vi "dataProcess_coherenceLength.vi"(0 "reference":refnum<class "OSA.lvclass">, 1 "samplesPerRefPeriod":i32, 2 "interferogram":sgl[](array[numeric]), 3 "X min interferogram (cm)":sgl, 4 "X max interferogram (cm)":sgl, 5 "error in (no error)":errorcluster, 6 "X range":T1(ring), 8 "X min (cm)":sgl format="%.2f", 10 "X max (cm)":sgl format="%.2f") -> (14 "duplicate reference":refnum<class "OSA.lvclass">, 15 "coherence length error(cm)":dbl, 16 "coherence length (cm)":dbl, 19 "error out":errorcluster)   [LabVIEW 2010, in "OSA.lvclass"]
doc: "Estimates the coherence length of the input light source by analyzing the interferogram.\n\nThis vi calls FTS_CoherenceLength_Array, (FTSLib.dll), with the interferogram input parameter pointing to the interferogram control data of this vi or, if empty, to the labview interferogram buffer. \n\nSee buffer_get.vi or trace_toLVBuffer.vi for OSA200 labview buffer handling."
uses:
  OSA.lvclass
  FTSLib.dll
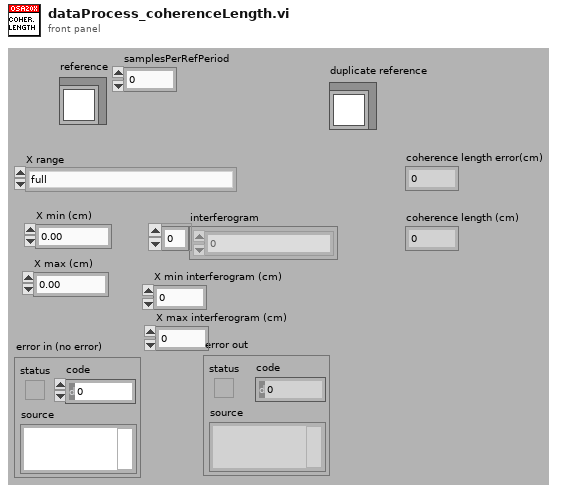
[diagram p1: front panel]
types:
  T1 = enum16{"full", "zero symmetric (-X min .... +X min)", "zero asymmetric (X min .... X max)"}
  T2 = cluster{"length":u32, "X min (cm)":sgl, "X max (cm)":sgl, "saturated":bool, "broadband":bool, "isMonoChromatic":bool, "peakToPeak, (counts)":dbl, "peakToPeak position (cm)":dbl, "samplesPerRefPeriod":i32}
  T3 = enum16{"get", "init", "set interferogram", "set spectrum", "cleanUp"}
  T4 = typedef "OSA.lvclass/ObjectAttributes.ctl" = cluster{"Stop":bool, "dataType":T5, "spectrometerIdx":u16, "buffer size interferogram":i32, "interferogram":cluster{"new":bool, "plot_x_ min":sgl, "plot_x_max":sgl, "plot_y_min":sgl, "plot_y_max":sgl, "Graph Intrfrgrm":T6, "timeStamp":u32, "signal (%)":dbl, "traces":cluster{"idx":u32, "broadBand":bool, "monoChromatic":bool, "peakToPeakSignal":dbl, "peakToPeakPos":dbl}[], "traces idx last":i32}, "spectrum":cluster{"new":bool, "plot_x_min":sgl, "plot_x_max":sgl, "plot_unit_x":T7, "plot_unit_y":T8, "plot_y_min":sgl, "plot_y_max":sgl, "Graph Spectrum":T6, "timeStamp":u32, "X_VAL_OPTIONS":enum16{"MIN_MAX", "ARRAY"}, "traces":cluster{"idx":u32}[], "traces idx last":i32}, "Thorlabs_OSA_64.lvclass:queue_action.ctlqueue ref":refnum<queue>, "action":T9, "plot zoom step":dbl, "buffer semaphore":T10, "acq stopped":bool, "dataType active":T5, "temperature (degr C)":sgl, "pressure (hPa)":sgl, "rel humidity (%)":sgl, "settings":cluster{"resolution":T11, "sensitivity":T12, "Average":bool, "average nr":u32, "apodisation":T13, "acq delay (ms)":u32, "airMesure":T14, "wmtr on":bool, "intfgrm_smooth_width":u16, "intfgrm_smooth_nrOfPasses":u16, "intfgrm_smooth":T15, "phaseCorrection":T16, "zeroFill":u8, "spectr_smooth":T15, "spectr_smooth_width":u16, "spectr_smooth_nrOfPasses":u16, "resolution (/cm)":sgl, "REF wavelength, (nm)":dbl, "gain_idx":u16, "gainAuto":bool, "gain_relative":dbl, "PD sensitivity mode":T17, "PD senseMode implemented":bool, "SensorTemperature implemented":bool, "SensorPressure implemented":bool, "SensorHumidity implemented":bool}, "peaks position":sgl[], "peaks width":sgl[], "peaks height":sgl[], "peaks max nr":u32, "peaks latest nr":i32, "peaks new":bool, "power":dbl, "power new":bool, "path":string, "wavelength (WNr)":dbl, "wavelength new":bool, "buffer size spectrum":i32, "status":string, "VI reference":refnum<vi>, "funcPointer":u64, "libraryPointer":u64, "singleAcquisition":bool, "coherenceLength (cm)":dbl, "coherenceLength new":bool, "spectrometer model":string, "spectrometer serial nr":string, "peaks thld left":sgl[], "peaks thld right":sgl[], "coherenceLength error (cm)":dbl, "ADC bits":u16, "peaks position centroid":sgl[], "peaks height centroid":sgl[], "OSA series":T18, "channel index (all)":u16}
  T5 = typedef "OSA.lvclass/acq_dataType.ctl" = enum16{"none", "interferogram", "spectrum"}
  T6 = typedef "OSA.lvclass/graph_intensity.ctl" = refnum<vi>
  T7 = typedef "OSA.lvclass/spectrum_x_unit.ctl" = enum16{"wavenr/cm", "THz", "eV", "nm_air", "nm_vac"}
  T8 = typedef "OSA.lvclass/y_unit.ctl" = enum16{"ADC counts", "dBm pwr absolute", "dBm pwr density", "mW pwr absolute", "mW pwr density"}
  T9 = typedef "OSA.lvclass/queue_action.ctl" = enum16{"none", "stop", "GUI_plotInterferogram", "GUI_plotSpectrum", "GUI_plotInterferogramRescale", "GUI_plotSpectrumRescale", "GUI_plotInterferogramReset", "GUI_plotSpectrumReset", "GUI_plotInterferogramAutoScaleY", "GUI_plotSpectrumAutoScaleY", "GUI_plotInterferogramZoomOut", "GUI_plotSpectrumZoomOut", "GUI_plotInterferogramPane", "GUI_plotSpectrumPane", "GUI_plotInterferogramZoomMouse", "GUI_plotSpectrumZoomMouse", "ENVIRONMENT temperature", "ENVIRONMENT pressure", "MODE_resolution set", "MODE_resolution get", "MODE_sensitivity set", "MODE_sensitivity get", "MODE_PDTemperature set", "MODE_PDTemperature get", "REBOOT/RESET firmware", "ACQASYNC_acquireSingleSpectrum", "ACQASYNC_continuous start", "ACQASYNC_continuous stop\n", "ACQASYNC_get last interferogram", "ACQASYNC_get last spectrum", "ACQASYNC_get last waveNr", "ACQOPT_interferogram smoothing set", "ACQOPT_interferogram smoothing get", "ACQOPT_spectrum smoothing set", "ACQOPT_spectrum smoothing get", "ACQOPT_apodisation type set", "ACQOPT_apodisation type get", "ACQOPT_phase correction type set", "ACQOPT_phase correction type get", "ACQOPT_acqIntervall_set", "ACQOPT_acqIntervall_get", "ACQOPT_average spectrum set", "ACQOPT_average spectrum get", "ACQOPT_rolling average set", "ACQOPT_rolling average get", "ACQOPT_zero fill factor set", "ACQOPT_zero fill factor get", "ACQOPT_cycle counting set", "ACQOPT_cycle counting get", "ACQOPT_air measure option set", "ACQOPT_air measure option get", "ACQOPT_gainLevel auto get", "ACQOPT_gainLevel auto set", "ACQOPT_gainLevel get", "ACQOPT_gainLevel set", "ACQOPT_getAll", "INSTRUMENT_PROPERTY_range_WaveNr_min", "INSTRUMENT_PROPERTY_range_WaveNr_max", "INSTRUMENT_PROPERTY_reference_wavelength_cm^-1", "INSTRUMENT_PROPERTY_samplesPerRefPeriod", "INSTRUMENT_PROPERTY_resolution_waveNrPercm", "INSTRUMENT_PROPERTY_availableGainLevels", "INSTRUMENT_PROPERTY_status", "CONVERT", "ANALYSE_POWER", "ANALYSE_PEAKS", "ANALYSE_WAVELENGTH", "ANALYSE_SPECTRUM", "ANALYSE_INTERFEROGRAM", "ANALYSE_COHERENCE_LENGTH", "MATH", "MATH_power", "MATH_peaks", "FILE", "miscellaneous"}
  T10 = typedef "Semaphore RefNum" = refnum<k1>
  T11 = typedef "OSA.lvclass/resolution.ctl" = enum16{"low", "high"}
  T12 = typedef "OSA.lvclass/sensitivityMode.ctl" = enum16{"low", "low medium", "high medium", "high"}
  T13 = typedef "OSA.lvclass/apodisation.ctl" = enum16{"NONE", "NORTON_BEER_WEAK", "NORTON_BEER_MEDIUM", "NORTON_BEER_STRONG", "TRIANGULAR", "COSINE", "HANN", "HAMMING", "BLACKMANHARRIS3", "BLACKMANHARRIS4", "GAUSSIAN"}
  T14 = typedef "OSA.lvclass/airMeasure.ctl" = enum16{"TEMPERATURE", "PRESSURE"}
  T15 = typedef "OSA.lvclass/smoothing.ctl" = enum16{"NONE", "BINOMIAL", "SAVITSKY_GOLAY", "FOURIER", "MOVING_AVERAGE", "GAUSSIAN"}
  T16 = typedef "OSA.lvclass/phaseCorrection.ctl" = enum16{"NONE", "MERTZ", "FORMAN", "MERTZ_FILE", "FORMAN_FILE", "FUTURE COMP."}
  T17 = typedef "OSA.lvclass/PDTemperatureMode.ctl" = enum16{"cool: better sensitivity/noise floor", "warm: extended wl range"}
  T18 = typedef "OSA_series.ctl" = enum16{"OSA200", "OSA300", "UNKNOWN"}
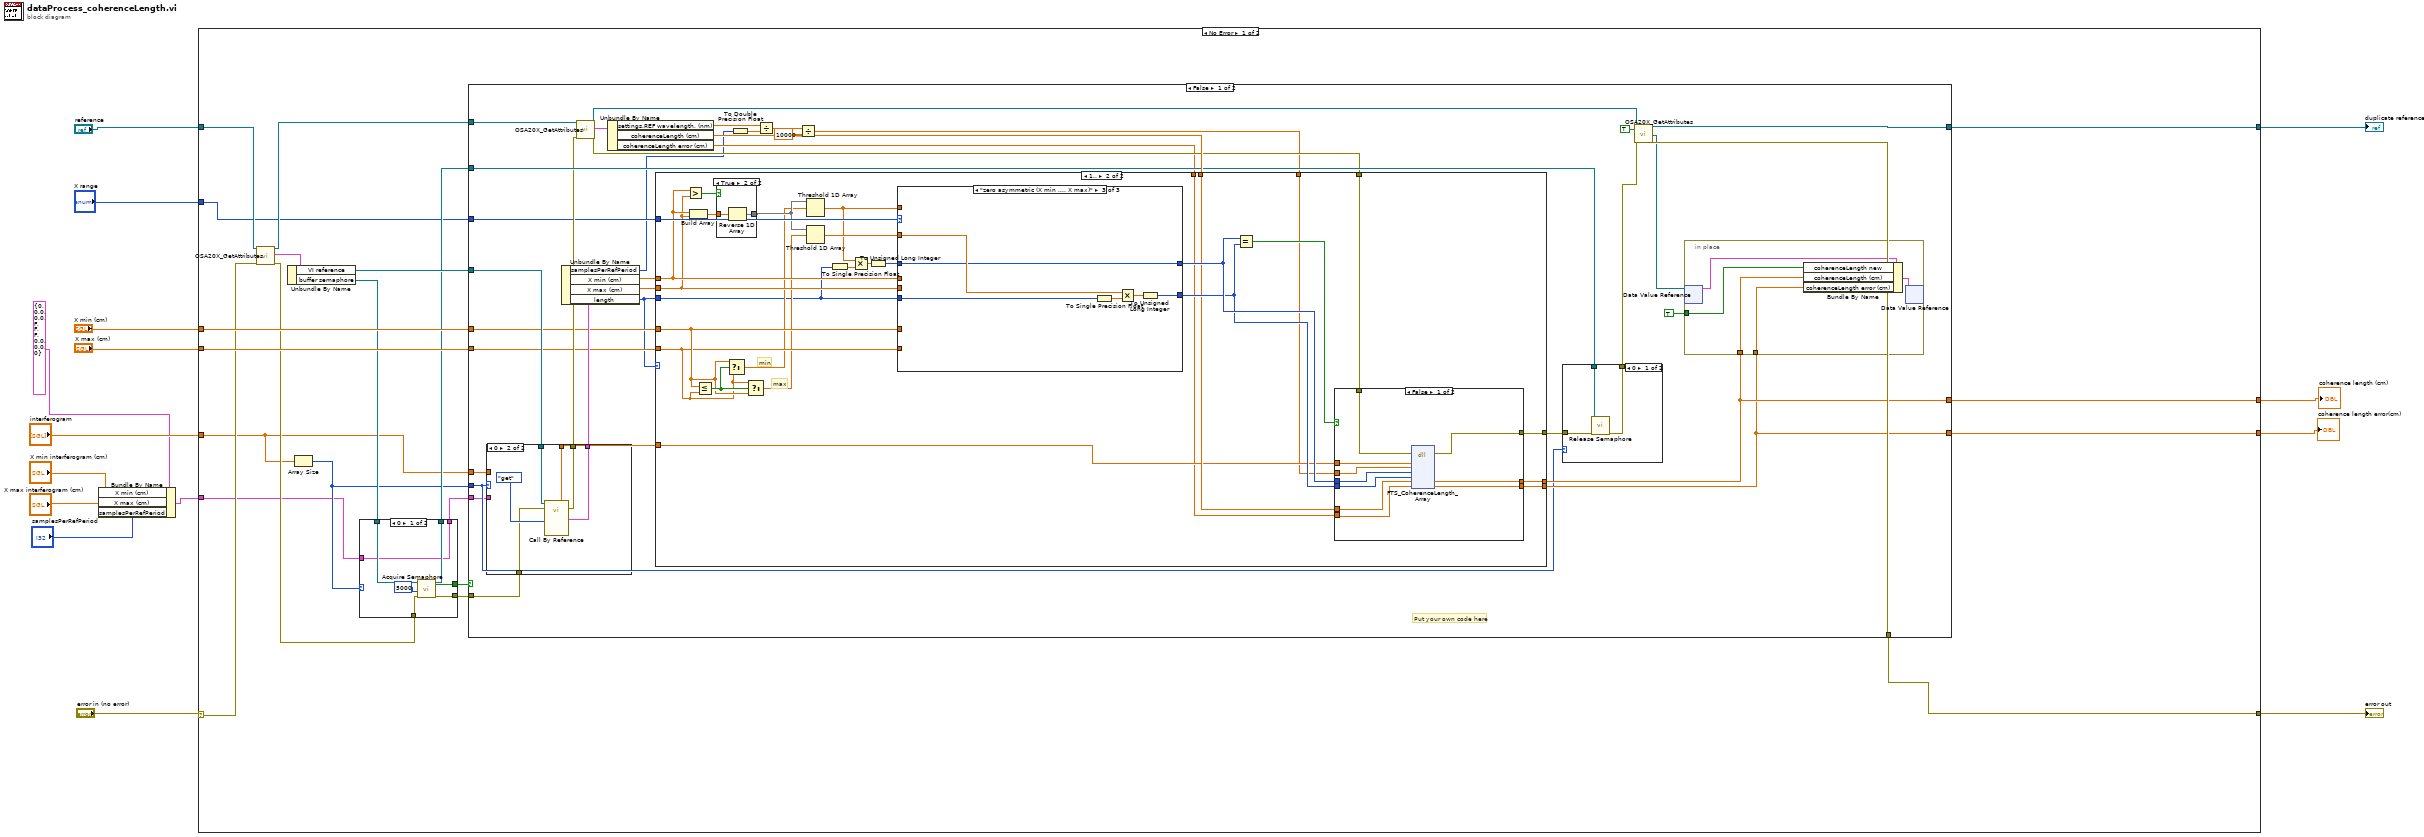
[diagram p0: block diagram]
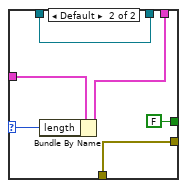
[diagram p2: hidden frame]
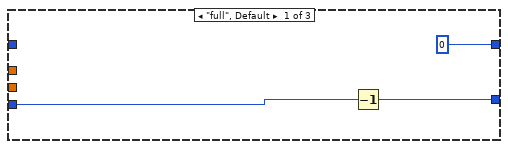
[diagram p7: hidden frame]
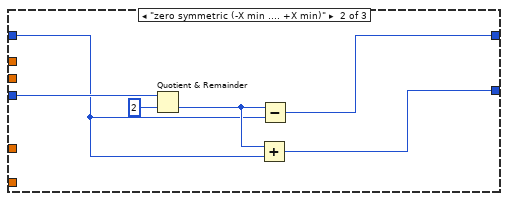
[diagram p8: hidden frame]
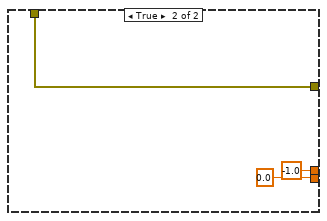
[diagram p9: hidden frame]
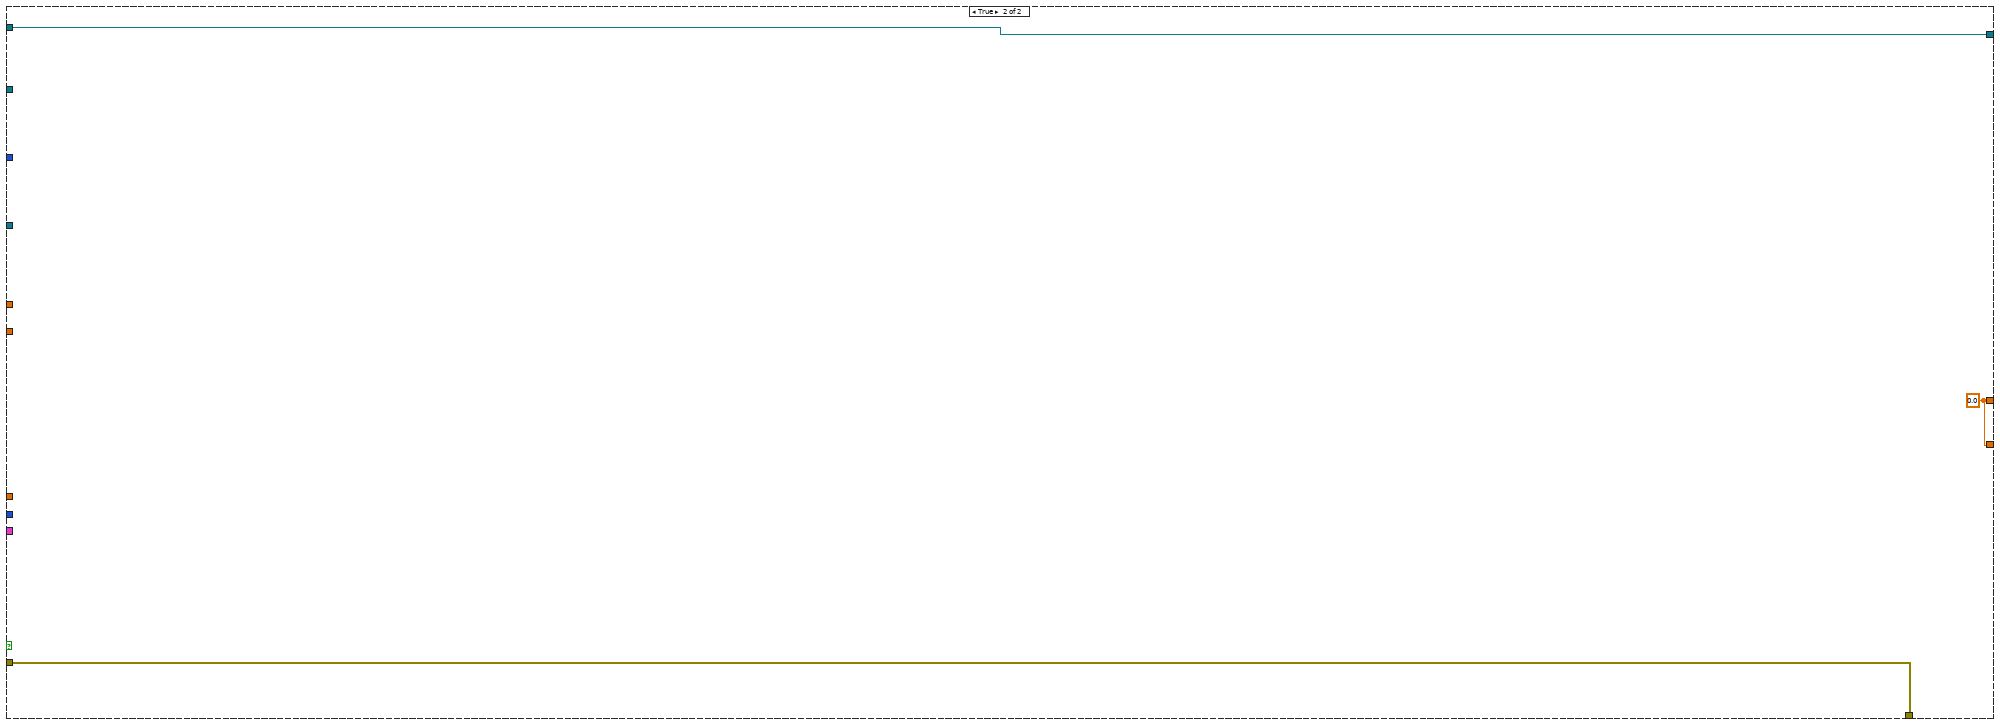
[diagram p10: hidden frame]
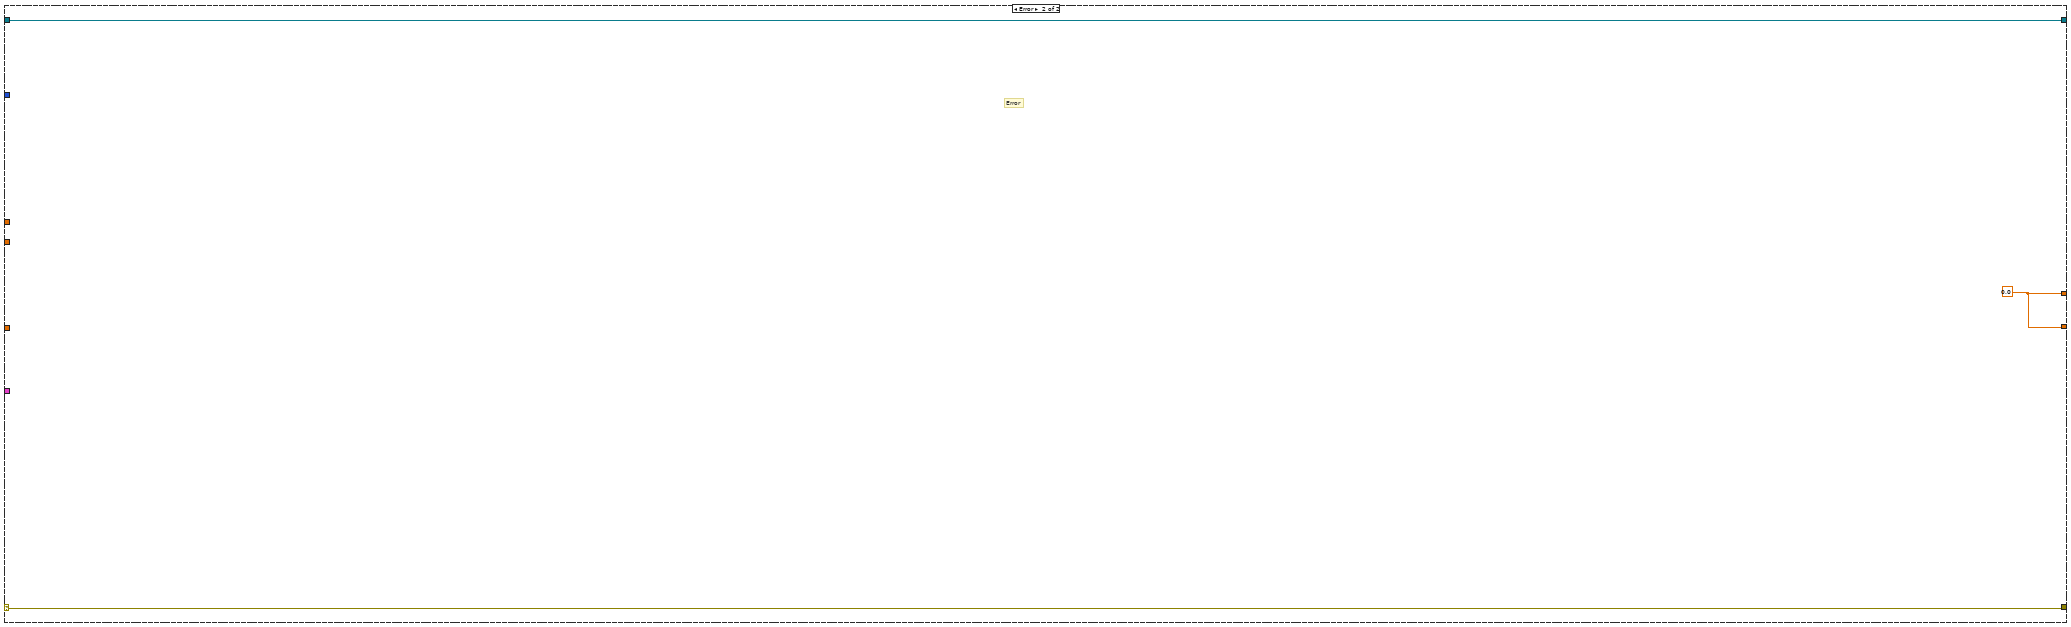
[diagram p11: hidden frame]
diagram:
  n1 = Bundle By Name(cluster=T2 {"length"=0, "X min (cm)"=0.0, "X max (cm)"=0.0, "saturated"=FALSE, "broadband"=FALSE, "isMonoChromatic"=FALSE, "peakToPeak, (counts)"=0.0, "peakToPeak position (cm)"=0.0, "samplesPerRefPeriod"=0} ("interferogram prop set"), "X min (cm)"="X min interferogram (cm)", "X max (cm)"="X max interferogram (cm)", "samplesPerRefPeriod"="samplesPerRefPeriod") -> (w5:T2)
  n2 = case shown="No Error" "error in (no error)" {
    selector: "error in (no error)" -> [w32 w170]
    tunnel: [w35 w170] -> w15
    tunnel: "reference" -> [w26 w171]
    tunnel: [w36 w171] -> w12
    tunnel: "X min (cm)" -> [w34 _]
    tunnel: "X max (cm)" -> [w33 _]
    tunnel: "X range" -> [w22 _]
    tunnel: [w21 w169] -> w8
    tunnel: [w20 w169] -> w7
    tunnel: "interferogram" -> [w19 _]
    tunnel: w5 -> [w17 _]
    frame No Error {
      n3 = call "OSA20X_GetAttributes.vi"("reference in"=w26, "error in (no error)"=w32) -> ("reference out"=w25:refnum<class "OSA.lvclass">, "Data"=w23:T4, "error out"=w31:errorcluster)  [unwired: 14 in, 1 out]
      n4 = Unbundle By Name(w23) -> ("VI reference"=w27:refnum<vi>, "buffer semaphore"=w29:T10)
      n5 = Array Size(array=w19) -> (size(s)=w18:i32)
      n6 = case shown="0" w18 {
        selector: w18 -> [_ w46]
        tunnel: w31 -> [w42 w48]
        tunnel: [w41 w48] -> w30
        tunnel: w29 -> [w40 w49]
        tunnel: [w39 FALSE ("timed out")] -> w28
        tunnel: [w38 w49] -> w24
        tunnel: w17 -> [w37 w45]
        tunnel: [w37 w44] -> w16
        frame 0 {
          n7 = call <vilib>:"Acquire Semaphore.vi"("error in (no error)"=w42, "ms timeout (-1)"=5000, "semaphore"=w40) -> ("error out"=w41:errorcluster, "timed out"=w39:bool, "semaphore out"=w38:T10)  [unwired: 2 in]
        }
        frame Default {
          n8 = Bundle By Name(cluster=w45, "length"=w46) -> (w44:T2)
        }
      }
      n9 = case shown="False" w28 {
        tunnel: w25 -> [w85 w168]
        tunnel: [w83 w168] -> w36
        tunnel: [w82 w167] -> w35
        tunnel: w34 -> [w61 _]
        tunnel: w33 -> [w60 _]
        tunnel: w30 -> [w80 w167]
        tunnel: w27 -> [w79 _]
        tunnel: w24 -> [w76 _]
        tunnel: w22 -> [w65 _]
        tunnel: [w58 w166] -> w21
        tunnel: [w57 w166] -> w20
        tunnel: w18 -> [w52 _]
        tunnel: w19 -> [w53 _]
        tunnel: w16 -> [w51 _]
        frame False {
          # "Put your own code here"
          n10 = case shown="0" w52 {
            tunnel: w80 -> [w91 w97]
            tunnel: w79 -> [_ w96]
            tunnel: [w91 w95] -> w75
            tunnel: [w92 w94] -> w69
            tunnel: [w90 w93] -> w64
            tunnel: w53 -> [w92 _]
            tunnel: w51 -> [w90 _]
            frame Default {
            }
            frame 0 {
              n11 = call-by-ref "?"(reference=w96, error in=w97, "action"=T3."get") -> (error out=w95:errorcluster, "interferogram"=w94:sgl[], "interferogram prop set"=w93:T2)  [unwired: 14 in, 4 out]
            }
          }
          n12 = Unbundle By Name(w64) -> ("samplesPerRefPeriod"=w50:i32, "X min (cm)"=w63:sgl, "X max (cm)"=w62:sgl, "length"=w59:u32)
          n13 = call "OSA20X_GetAttributes.vi"("reference in"=w85, "error in (no error)"=w75) -> ("reference out"=w84:refnum<class "OSA.lvclass">, "Data"=w73:T4, "error out"=w70:errorcluster)  [unwired: 14 in, 1 out]
          n14 = Unbundle By Name(w73) -> ("settings.REF wavelength, (nm)"=w68:dbl, "coherenceLength (cm)"=w81:dbl, "coherenceLength error (cm)"=w66:dbl)
          n15 = To Double Precision Float(number=w50) -> (double precision float=w67:dbl)
          n16 = Divide(x=w68, y=w67) -> (x/y=w56:dbl)
          n17 = Divide(x=w56, y=10000000.0) -> (x/y=w54:dbl)
          n18 = case shown="1.." w59 {
            tunnel: w81 -> [w100 w126]
            tunnel: [w99 w125] -> w78
            tunnel: w70 -> [w99 w124]
            tunnel: w69 -> [_ w123]
            tunnel: w54 -> [_ w122]
            tunnel: [w100 w121] -> w58
            tunnel: [w101 w120] -> w57
            tunnel: w66 -> [w101 w119]
            tunnel: w65 -> [_ w118]
            tunnel: w63 -> [_ w114]
            tunnel: w62 -> [_ w113]
            tunnel: w61 -> [_ w111]
            tunnel: w60 -> [_ w110]
            tunnel: w59 -> [_ w104]
            frame 0, Default {
            }
            frame 1.. {
              # "max"
              # "min"
              n19 = Greater?(x=w114, y=w113) -> (0:w116:bool)
              n20 = Build Array(w114, w113) -> (w117:sgl[])
              n21 = Less Or Equal?(x=w111, y=w110) -> (x <= y?=w112:bool)
              n22 = case shown="True" w116 {
                tunnel: w117 -> [w130 w132]
                tunnel: [w130 w131] -> w115
                frame False {
                }
                frame True {
                  n23 = Reverse 1D Array(array=w132) -> (reversed array=w131:sgl[])
                }
              }
              n24 = Select(t=w111, s=w112, f=w110) -> (s? t:f=w109:sgl)
              n25 = Select(t=w110, s=w112, f=w111) -> (s? t:f=w108:sgl)
              n26 = Threshold 1D Array(2:w109, 3:w115) -> (0:w105:sgl)  [unwired: 1 in]
              n27 = Threshold 1D Array(2:w108, 3:w115) -> (0:w107:sgl)  [unwired: 1 in]
              n28 = To Single Precision Float(number=w104) -> (single precision float=w106:sgl)
              n29 = Multiply(x=w105, y=w106) -> (x*y=w103:sgl)
              n30 = To Unsigned Long Integer(number=w103) -> (unsigned 32bit integer=w102:u32)
              n31 = case shown="\"zero asymmetric (X min .... X max)\"" w118 {
                tunnel: w111 -> [_ _ _]
                tunnel: w110 -> [_ _ _]
                tunnel: [u32 0 w137 w142] -> w129
                tunnel: [w134 w136 w145] -> w128
                tunnel: w114 -> [_ _ _]
                tunnel: w113 -> [_ _ _]
                tunnel: w104 -> [w133 w141 w144]
                tunnel: w105 -> [_ _ _]
                tunnel: w107 -> [_ _ w143]
                tunnel: w102 -> [_ w138 w142]
                frame "full", Default {
                  n32 = Decrement(x=w133) -> (x-1=w134:u32)
                }
                frame "zero symmetric (-X min .... +X min)" {
                  n33 = Quotient & Remainder(x=w141, y=u32 2) -> (floor(x/y)=w139:u32)  [unwired: 1 out]
                  n34 = Add(x=w139, y=w138) -> (x+y=w136:u32)
                  n35 = Subtract(x=w139, y=w138) -> (x-y=w137:u32)
                }
                frame "zero asymmetric (X min .... X max)" {
                  n36 = To Single Precision Float(number=w144) -> (single precision float=w147:sgl)
                  n37 = Multiply(x=w143, y=w147) -> (x*y=w146:sgl)
                  n38 = To Unsigned Long Integer(number=w146) -> (unsigned 32bit integer=w145:u32)
                }
              }
              n39 = Equal?(x=w129, y=w128) -> (x = y?=w127:bool)
              n40 = case shown="False" w127 {
                tunnel: w126 -> [w152 _]
                tunnel: w123 -> [w155 _]
                tunnel: w129 -> [w154 _]
                tunnel: w128 -> [w153 _]
                tunnel: [w156 w160] -> w125
                tunnel: w124 -> [w157 w160]
                tunnel: w122 -> [w151 _]
                tunnel: [w150 -1.0 ("coherenceLength")] -> w121
                tunnel: [w149 0.0 ("coherenceLength_error")] -> w120
                tunnel: w119 -> [w148 _]
                frame False {
                  n41 = dll-call lib="FTSLib.dll" fn="FTS_CoherenceLength_Array"(error in=w157, "intrfgrm"=w155, "sampleDist_cm"=w151, "idxStart"=w154, "idxStop"=w153, "coherenceLength"=w152, "coherenceLength_error"=w148) -> (error out=w156:errorcluster, "coherenceLength"=w150:dbl, "coherenceLength_error"=w149:dbl)  [unwired: 7 in, 1 out]
                }
                frame True {
                }
              }
            }
          }
          n42 = case shown="0" w52 {
            tunnel: w78 -> [w88 w89]
            tunnel: [w87 w89] -> w77
            tunnel: w76 -> [w86 _]
            frame 0 {
              n43 = call <vilib>:"Release Semaphore.vi"("error in (no error)"=w88, "semaphore"=w86) -> ("error out"=w87:errorcluster)  [unwired: 4 in, 1 out]
            }
            frame Default {
            }
          }
          n44 = call "OSA20X_GetAttributes.vi"("reference in"=w84, "OnlyGetDvrReference(False)"=TRUE, "error in (no error)"=w77) -> ("reference out"=w83:refnum<class "OSA.lvclass">, "DataRef"=w72:refnum<data-value>, "error out"=w82:errorcluster)  [unwired: 13 in, 1 out]
          n45 = in-place {
            in-place-border: TRUE ("peaks new") -> [w164]
            in-place-border: w58 -> [w162]
            in-place-border: w57 -> [w161]
            n46 = in-place-dvr #1(w72) -> (w165:T4)  [unwired: 1 out]
            n47 = Bundle By Name(cluster=w165, "coherenceLength new"=w164, "coherenceLength (cm)"=w162, "coherenceLength error (cm)"=w161) -> (w163:T4)
            n48 = in-place-dvr #1(w163) -> ()  [unwired: 2 out]
          }
        }
        frame True {
          w166 = 0.0 ("coherenceLength")
        }
      }
    }
    frame Error {
      w169 = 0.0 ("coherenceLength")
      # "Error"
    }
  }
  "error out" <- w15
  "duplicate reference" <- w12
  "coherence length error(cm)" <- w7
  "coherence length (cm)" <- w8
